vi "Read groupName.vi"(8 "error in":errorcluster, 11 "group configuration in":refnum<class "group configuration.lvclass">) -> (0 "error out":errorcluster, 2 "groupName":string, 3 "group configuration out":refnum<class "group configuration.lvclass">)   [LabVIEW 2013, in "group configuration.lvclass"]
uses:
  group configuration.lvclass
  CEF_TreeControl/serializable configuration/NISE_CEF_serializable configuration.lvclass
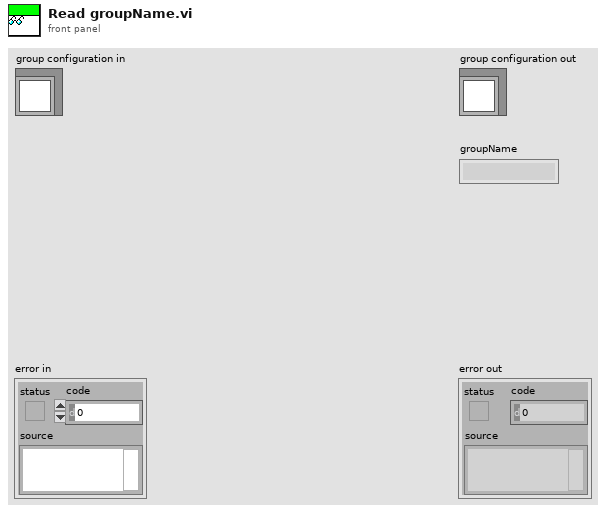
[diagram p1: front panel]
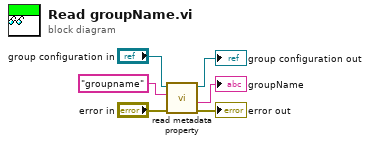
[diagram p0: block diagram]
diagram:
  n1 = call "read metadata property.vi"("error in"="error in", "key"="groupname", "configuration in"="group configuration in") -> ("error out"=→"error out":errorcluster, "value"=→"groupName":string, "configuration out"=→"group configuration out":refnum<class "group configuration.lvclass">)  [unwired: 5 in, 1 out]
